vi "String to IMAQ.vi"(8 "Error In":errorcluster, 11 "Input Image String":string) -> (0 "Error Out":errorcluster, 3 "Image":T1(plugin-control))   [LabVIEW 2014]
uses:
  <vilib>/vision/Image Controls.llb/IMAQ Image.ctl
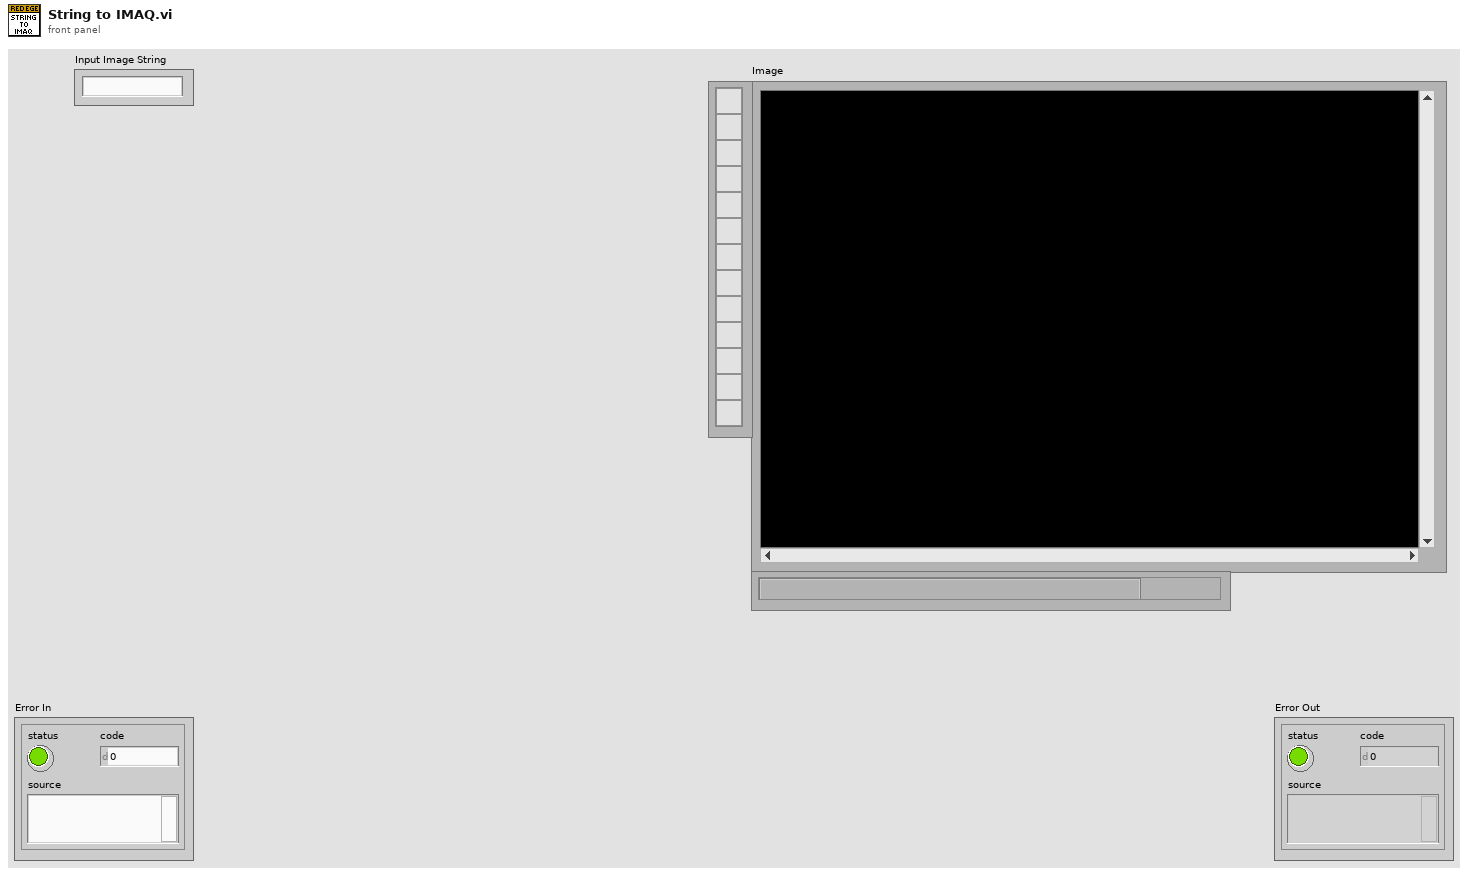
[diagram p1: front panel]
types:
  T1 = typedef "IMAQ Image.ctl" = refnum<image>
  T2 = typedef "Image Type" = u32
  T3 = typedef "imagedata.ctl" = cluster{"image type":i32, "image depth":i32, "image":u8[], "mask":u8[], "colors":u32[], "Rectangle":cluster{"left":i16, "top":i16, "right":i16, "bottom":i16}}
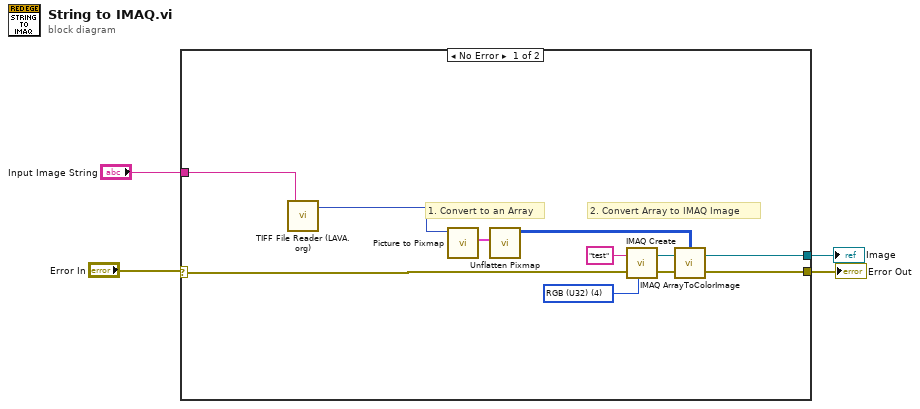
[diagram p0: block diagram]
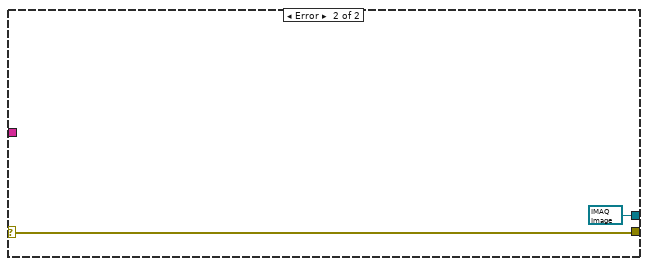
[diagram p2: hidden frame]
diagram:
  n1 = case shown="No Error" "Error In" {
    selector: "Error In" -> [w8 w17]
    tunnel: "Input Image String" -> [w9 _]
    tunnel: [w6 w17] -> w2
    tunnel: [w5 T1 refnum ("Image Out")] -> w1
    frame No Error {
      w12 = T2 4 items=["Grayscale (U8)", "Grayscale (I16)", "Grayscale (SGL)", "Complex (CSG)", "RGB (U32)", "HSL (U32)", "RGB (U64)", "Grayscale (U16)"] ("Image Type")
      # "2. Convert Array to IMAQ Image"
      # "1. Convert to an Array"
      n2 = call "TIFF File Reader (LAVA.org).vi"("Input Image"=w9) -> ("Grayscale"=w10:picture)  [unwired: 3 in, 3 out]
      n3 = call <vilib>:"Picture to Pixmap.vi"("picture"=w10) -> ("image data"=w15:T3)  [unwired: 9 in, 1 out]
      n4 = call <vilib>:"Unflatten Pixmap.vi"("image data"=w15) -> ("24-bit pixmap"=w11:u32[][])  [unwired: 4 in, 6 out]
      n5 = call "IMAQ Create"("Image Name"="test", "Image Type"=w12, "error in (no error)"=w8) -> ("New Image"=w14:T1, "error out"=w7:errorcluster)  [unwired: 2 in]
      n6 = call "IMAQ ArrayToColorImage"("Image Pixels (U32)"=w11, "Image"=w14, "error in (no error)"=w7) -> ("Image Out"=w5:T1, "error out"=w6:errorcluster)  [unwired: 2 in]
    }
    frame Error {
    }
  }
  "Error Out" <- w2
  "Image" <- w1
